vi "Free.vi"(8 "error in (no error)":errorcluster, 11 "modbus in":refnum<class "libmodbus.lvclass">) -> (0 "error out":errorcluster)   [LabVIEW 2017, in "libmodbus.lvlib" / "libmodbus.lvclass"]
doc: "Frees the libmodbus context."
uses:
  libmodbus.lvclass
  libmodbus.lvclass/libmodbus.ctl
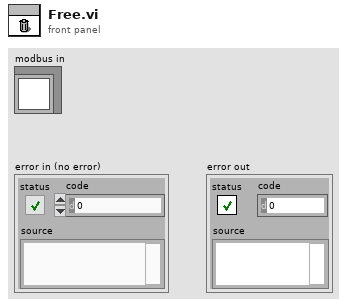
[diagram p1: front panel]
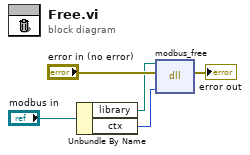
[diagram p0: block diagram]
diagram:
  n1 = Unbundle By Name("modbus in") -> ("library"=w3:path, "ctx"=w4:i64)
  n2 = dll-call lib="?" fn="modbus_free"(path in=w3, error in="error in (no error)", "ctx"=w4) -> (error out=→"error out":errorcluster)  [unwired: 3 in, 1 out]
